vi "Parameters.vi"(8 "error in (no error)":errorcluster, 11 "Parametrized Test Case Test Double In":refnum<class "Parametrized Test Case Test Double.lvclass">) -> (0 "error out":errorcluster, 2 "Parameters":T1(array[cluster]))   [LabVIEW 2020, in "Parametrized Test Case Test Double.lvclass"]
uses:
  Parametrized Test Case Test Double.lvclass
  C:/git/astemes-lunit-parameterized-test/source/Parameterized Test Case/Parameterized Test Case.lvclass
  Parametrized Test Case Test Double.lvclass/Parametrized Test Case Test Double.ctl
  C:/Program Files (x86)/National Instruments/LabVIEW 2020/vi.lib/Astemes/LUnit/Test Case.lvclass
  C:/Program Files (x86)/National Instruments/LabVIEW 2020/vi.lib/Astemes/LUnit/LUnit Runnable.lvclass
  C:/git/astemes-lunit-parameterized-test/source/Parametrized Test Case Test Double/Parametrized Test Case Test Double.lvclass
  Parameterized Test Case/Parameterized Test Case.lvclass
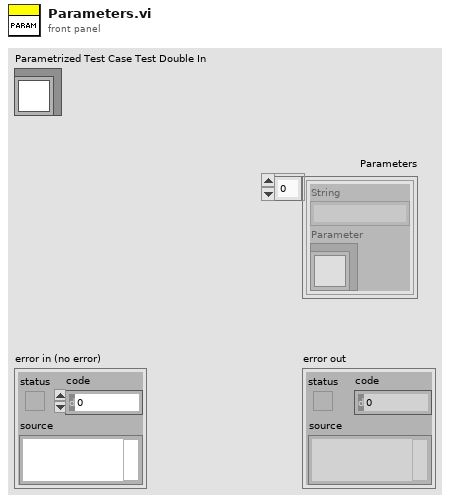
[diagram p1: front panel]
types:
  T1 = cluster{"String":string, "Parameter":refnum<class "Parameterized Test Case.lvclass">}[]
  T2 = cluster{"String":string, "Parametrized Test Case Test Double.lvclass":refnum<class "Parametrized Test Case Test Double.lvclass">}
  T3 = cluster{"String":string, "Parametrized Test Case Test Double.lvclass":refnum<class "Parametrized Test Case Test Double.lvclass">}[]
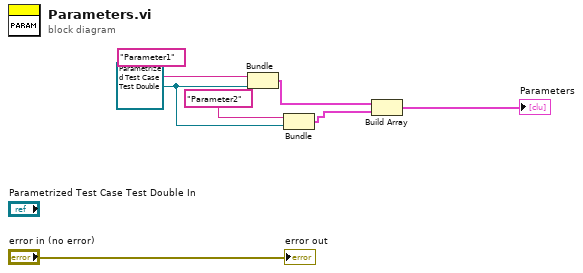
[diagram p0: block diagram]
diagram:
  w4 = refnum<class "Parametrized Test Case Test Double.lvclass"> refnum ("Parametrized Test Case Test Double.lvclass")
  n1 = Bundle("String"="Parameter1", "Parametrized Test Case Test Double.lvclass"=w4) -> (w3:T2)  [unwired: 1 in]
  n2 = Bundle("String"="Parameter2", "Parametrized Test Case Test Double.lvclass"=w4) -> (w2:T2)  [unwired: 1 in]
  n3 = Build Array(w3, w2) -> (→"Parameters":T3)
  "error out" <- "error in (no error)"
